vi "checkIncomingAgent.vi"(0 "Host_Reference":refnum<class "HGF_Reference.lvclass">, 2 "timeout in ms (-1)":i32, 3 "MoAgSy_Message":refnum<class "MoAgSy_Message.lvclass">, 5 "error in (no error)":errorcluster) -> (14 "dup Host_Reference":refnum<class "HGF_Reference.lvclass">, 16 "dup timeout in ms (-1)":i32, 17 "dup MoAgSy_Message":refnum<class "MoAgSy_Message.lvclass">, 18 "start agent?":bool=TRUE, 19 "error out":errorcluster)   [LabVIEW 2009, in "MoAgSy.lvlib" / "MoAgSy_Host.lvclass"]
doc: "<B>public</B> VI checks incoming Agents before they are started.\nIf an Agent is blacklisted, start is refused. If whitelisted, VI checks if Host is full,\nif unlisted, Host settings determine what to do. <B>unlisted not yet implemented</B>\nReply Message will be send by this VI, too.\n\nF.Berck@gsi.de\nGSI Darmstadt 2009"
uses:
  MoAgSy_Host.lvclass
  HGF_BaseClasses/HGF_Reference/HGF_Reference.lvclass
  MoAgSy_Message/MoAgSy_Message.lvclass
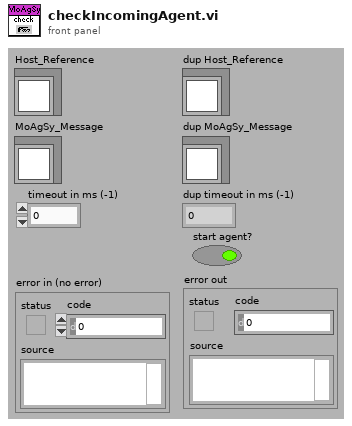
[diagram p1: front panel]
types:
  T1 = enum16{"Not a visitable", "Agent blacklisted", "Host full", "ok"}
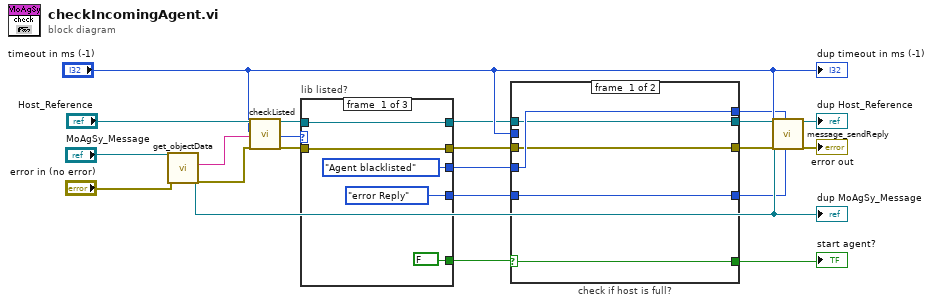
[diagram p0: block diagram]
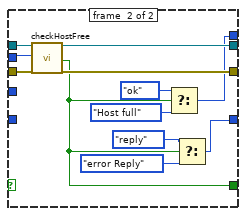
[diagram p2: hidden frame]
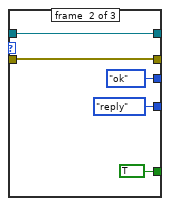
[diagram p3: hidden frame]
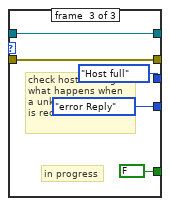
[diagram p4: hidden frame]
diagram:
  n1 = call "get_objectData.vi"("MoAgSy_Message.lvclass in"="MoAgSy_Message", "error in (no error)"="error in (no error)") -> ("MoAgSy_Message.lvclass out"=w12:refnum<class "MoAgSy_Message.lvclass">, "Object Library"=w21:string, "error out"=w19:errorcluster)  [unwired: 15 out]
  "dup MoAgSy_Message" <- w12
  n2 = call "checkListed.vi"("Host_Reference"="Host_Reference", "timeout in ms (-1)"="timeout in ms (-1)", "Library"=w21, "error in (no error)"=w19) -> ("dup Host_Reference"=w16:refnum<class "HGF_Reference.lvclass">, "listed?"=w17:enum16{"blacklisted", "whitelisted", "unlisted"}, "error out"=w15:errorcluster)  [unwired: 13 out]
  n3 = case "lib listed?" shown="\"unlisted\"" w17 {
    tunnel: w16 -> [w25 w31 w37]
    tunnel: w15 -> [w26 w32 w36]
    tunnel: [FALSE ("start agent?") TRUE ("start agent?") FALSE ("start agent?")] -> w11
    tunnel: [w26 w32 w36] -> w2
    tunnel: [w25 w31 w37] -> w4
    tunnel: [enum16{"error Reply", "reply"}."error Reply" ("Message Type") enum16{"error Reply", "reply"}."reply" ("Message Type") enum16{"error Reply", "reply"}."error Reply" ("Message Type")] -> w9
    tunnel: [T1."Agent blacklisted" ("message") T1."ok" ("message") T1."Host full" ("message")] -> w6
    frame #0 {
    }
    frame #1 {
    }
    frame #2 {
      # "check host settings\nwhat happens when\na unknown agent\nis received?"
      # "in progress"
    }
  }
  n4 = case "check if host is full?" shown="True" w11 {
    selector: w11 -> [w42 _]
    tunnel: [w42 w43] -> w10
    tunnel: w9 -> [w41 _]
    tunnel: [w41 w49] -> w8
    tunnel: w6 -> [w40 _]
    tunnel: [w40 w44] -> w5
    tunnel: w4 -> [w39 w54]
    tunnel: [w39 w53] -> w3
    tunnel: w2 -> [w38 w52]
    tunnel: [w38 w51] -> w1
    tunnel: "timeout in ms (-1)" -> [_ w50]
    frame #0 {
    }
    frame #1 {
      n5 = call "checkHostFree.vi"("Host_Reference"=w54, "timeout in ms (-1)"=w50, "error in (no error)"=w52) -> ("dup Host_Reference"=w53:refnum<class "HGF_Reference.lvclass">, "free4agents"=w43:bool, "error out"=w51:errorcluster)  [unwired: 14 out]
      n6 = Select(t=T1."ok" ("message"), s=w43, f=T1."Host full" ("message")) -> (s? t:f=w44:T1)
      n7 = Select(t=enum16{"error Reply", "reply"}."reply" ("Message Type"), s=w43, f=enum16{"error Reply", "reply"}."error Reply" ("Message Type")) -> (s? t:f=w49:enum16{"error Reply", "reply"})
    }
  }
  "start agent?" <- w10
  n8 = call "message_sendReply.vi"("Host_Reference"=w3, "MoAgSy_Message"=w12, "timeout in ms (-1)"="timeout in ms (-1)", "error in (no error)"=w1, "message"=w5, "Message Type"=w8) -> ("dup Host_Reference"=→"dup Host_Reference":refnum<class "HGF_Reference.lvclass">, "error out"=→"error out":errorcluster)  [unwired: 1 in, 11 out]
  "dup timeout in ms (-1)" <- "timeout in ms (-1)"
